vi "Read Characters with check.vi"(2 "Call EnFlo Error Handler?":bool=TRUE, 3 "file (use dialog)":path) -> (0 "error out":errorcluster, 1 "Read String":string)   [LabVIEW 2022 SP3]
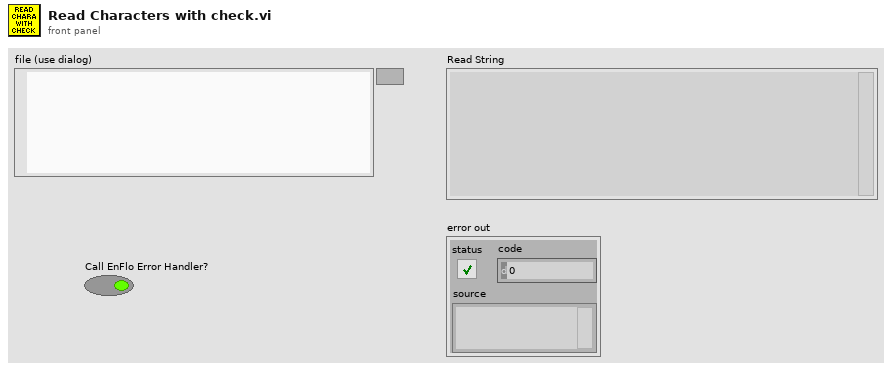
[diagram p1: front panel]
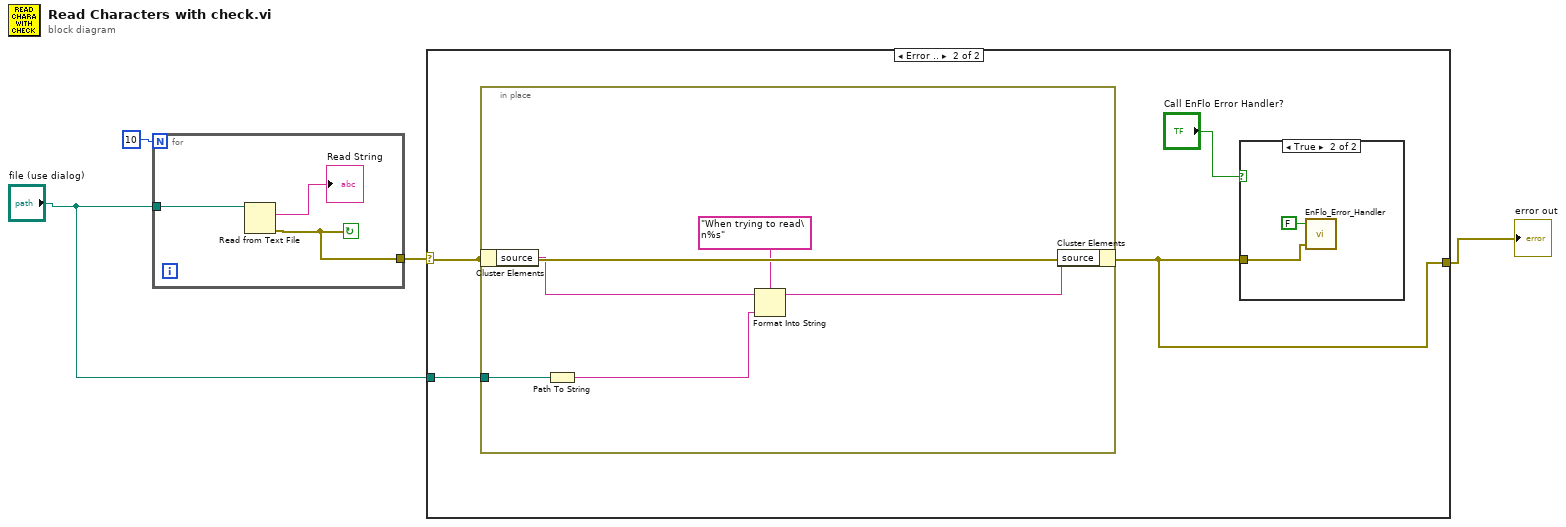
[diagram p0: block diagram]
diagram:
  n1 = for {
    N: 10 -> [_]
    tunnel: "file (use dialog)" -> [w7]
    tunnel: [w5] -> w3
    stop <- w5 continue-if-true
    n2 = Read from Text File(file (use dialog)=w7) -> (text=→"Read String":string, error out=w5:errorcluster)  [unwired: 3 in, 2 out]
  }
  n3 = case shown="Error .." w3 {
    selector: w3 -> [w8 w9]
    tunnel: [w8 w9] -> w2
    tunnel: "file (use dialog)" -> [_ w10]
    frame No Error {
    }
    frame Error {
      n4 = in-place {
        in-place-border: w10 -> [w16]
        n5 = in-place-cluster #1(w9) -> ("source"=w15:string)
        n6 = Path To String(path=w16) -> (string=w14:string)
        n7 = Format Into String(format string="When trying to read\n%s", initial string=w15, w14) -> (resulting string=w12:string)  [unwired: 1 in, 1 out]
        n8 = in-place-cluster #1("source"=w12) -> ()  [unwired: 1 out]
      }
      n9 = case shown="True" "Call EnFlo Error Handler?" {
        tunnel: w9 -> [_ w17]
        frame False {
        }
        frame True {
          n10 = call "EnFlo_Error_Handler.vi"("error in (no error)"=w17, "Dialog Box (F)"=FALSE) -> ()  [unwired: 2 in, 2 out]
        }
      }
    }
  }
  "error out" <- w2
